vi "TW_Base64Conversion.vi"(9 "Base64 String in":string, 11 "String":string) -> (0 "error out":errorcluster, 1 "String out":string, 3 "Base64 String":string)   [LabVIEW 2019]
panel:
  in  "error in (no error)":errorcluster
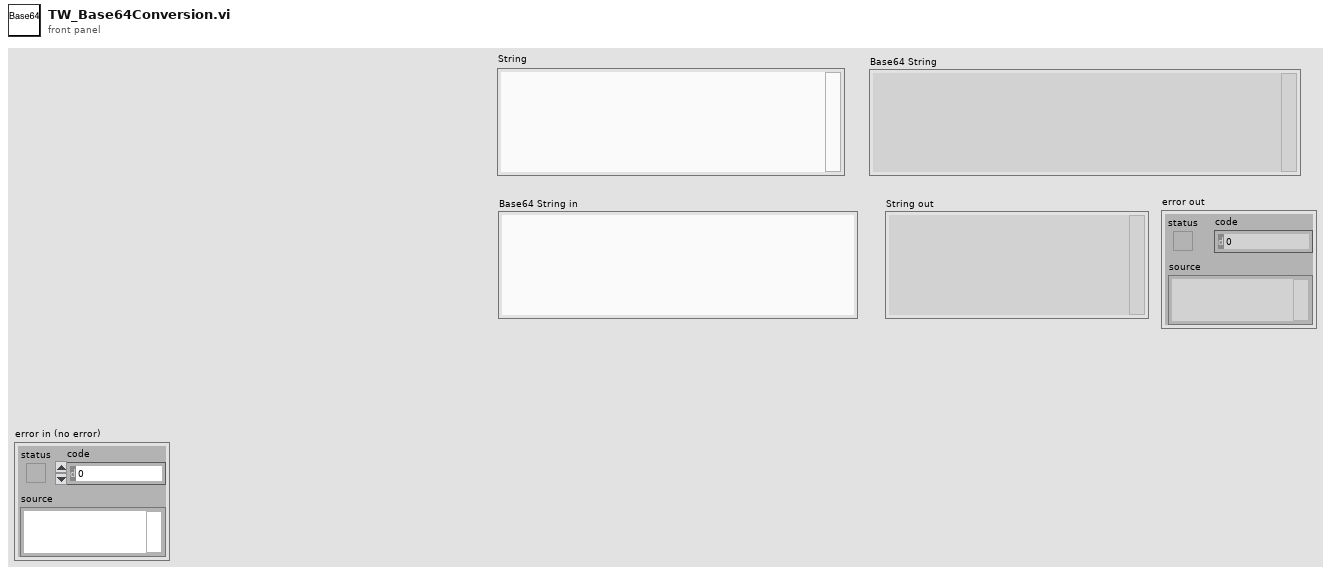
[diagram p1: front panel]
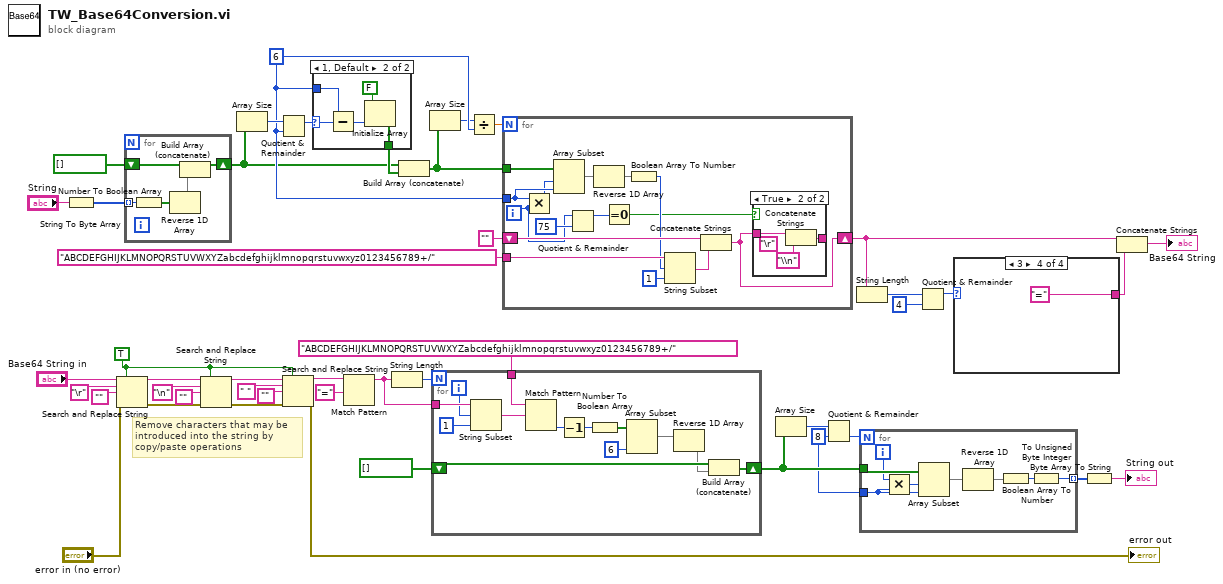
[diagram p0: block diagram]
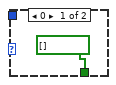
[diagram p2: hidden frame]
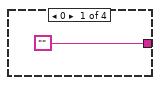
[diagram p3: hidden frame]
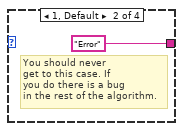
[diagram p4: hidden frame]
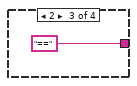
[diagram p5: hidden frame]
diagram:
  w1 = TRUE ("replace all? (F)")
  w18 = 8 ("y")
  w30 = 6 ("y")
  # "Remove characters that may be\nintroduced into the string by\ncopy/paste operations"
  n1 = String To Byte Array(string="String") -> (unsigned byte array=w44:u8[])
  n2 = Search and Replace String(replace all?=w1, input string="Base64 String in", search string="\r" ("replace string (\"\")"), replace string="", error in="error in (no error)") -> (result string=w11:string, error out=w9:errorcluster)  [unwired: 5 out]
  n3 = for {
    tunnel: w44 -> [w50] mode=indexing
    shift-right: [w47] -> w27
    shift-left: bool[] [] -> [w49]
    n4 = Number To Boolean Array(number=w50) -> (Boolean array=w48:bool[])
    n5 = Reverse 1D Array(array=w48) -> (reversed array=w46:bool[])
    n6 = Build Array (concatenate)(w49, w46) -> (w47:bool[])
  }
  n7 = Search and Replace String(replace all?=w1, input string=w11, search string="\n" ("replace string (\"\")"), replace string="", error in=w9) -> (result string=w5:string, error out=w4:errorcluster)  [unwired: 5 out]
  n8 = Array Size(array=w27) -> (size(s)=w33:i32)
  n9 = Quotient & Remainder(x=w33, y=w30) -> (x-y*floor(x/y)=w32:i32)  [unwired: 1 out]
  n10 = Search and Replace String(replace all?=w1, input string=w5, search string=" " ("replace string (\"\")"), replace string="", error in=w4) -> (result string=w2:string, error out=→"error out":errorcluster)  [unwired: 5 out]
  n11 = case shown="1, Default" w32 {
    selector: w32 -> [_ w55]
    tunnel: [bool[] [] w52] -> w31
    tunnel: w30 -> [_ w54]
    frame 0 {
    }
    frame 1, Default {
      n12 = Subtract(x=w54, y=w55) -> (x-y=w56:i32)
      n13 = Initialize Array(FALSE, w56) -> (w52:bool[])
    }
  }
  n14 = Match Pattern(string=w2, regular expression="=") -> (before substring=w23:string)  [unwired: 4 out]
  n15 = String Length(string=w23) -> (length=w26:i32)
  n16 = Build Array (concatenate)(w27, w31) -> (w29:bool[])
  n17 = Array Size(array=w29) -> (size(s)=w28:i32)
  n18 = for {
    N: w26 -> [_]
    tunnel: w23 -> [w69]
    tunnel: "ABCDEFGHIJKLMNOPQRSTUVWXYZabcdefghijklmnopqrstuvwxyz0123456789+/" -> [w66]
    shift-right: [w59] -> w19
    shift-left: bool[] [] -> [w58]
    i -> [w67]
    n19 = String Subset(string=w69, offset (0)=w67, length (rest)=1 ("length (rest)")) -> (substring=w65:string)
    n20 = Match Pattern(string=w66, regular expression=w65) -> (offset past match=w64:i32)  [unwired: 1 in, 3 out]
    n21 = Decrement(x=w64) -> (x-1=w63:i32)
    n22 = Number To Boolean Array(number=w63) -> (Boolean array=w62:bool[])
    n23 = Array Subset(array=w62, length=6) -> (w60:bool[])  [unwired: 1 in]
    n24 = Reverse 1D Array(array=w60) -> (reversed array=w57:bool[])
    n25 = Build Array (concatenate)(w58, w57) -> (w59:bool[])
  }
  n26 = Divide(x=w28, y=w30) -> (x/y=w34:dbl)
  n27 = for {
    N: w34 -> [_]
    tunnel: w29 -> [w84]
    tunnel: w30 -> [w83]
    tunnel: "ABCDEFGHIJKLMNOPQRSTUVWXYZabcdefghijklmnopqrstuvwxyz0123456789+/" -> [w82]
    shift-right: [w70] -> w36
    shift-left: "" -> [w80]
    i -> [w73]
    n28 = Multiply(x=w83, y=w73) -> (x*y=w74:i32)
    n29 = Array Subset(array=w84, index=w74, length=w83) -> (w76:bool[])
    n30 = Quotient & Remainder(x=w73, y=75) -> (x-y*floor(x/y)=w72:i32)  [unwired: 1 out]
    n31 = Reverse 1D Array(array=w76) -> (reversed array=w77:bool[])
    n32 = Equal To 0?(x=w72) -> (x = 0?=w71:bool)
    n33 = Boolean Array To Number(Boolean array=w77) -> (number=w78:u32)
    n34 = String Subset(string=w82, offset (0)=w78, length (rest)=1 ("length (rest)")) -> (substring=w79:string)
    n35 = Concatenate Strings(w80, w79) -> (w70:string)
    n36 = case shown="True" w71 {
      tunnel: w70 -> [w85 w87]
      tunnel: [w85 w88] -> _
      frame False {
      }
      frame True {
        (unwired) "\r"
        n37 = Concatenate Strings(w87, "\\n" ("string")) -> (w88:string)
      }
    }
  }
  n38 = Array Size(array=w19) -> (size(s)=w21:i32)
  n39 = Quotient & Remainder(x=w21, y=w18) -> (floor(x/y)=w20:i32)  [unwired: 1 out]
  n40 = String Length(string=w36) -> (length=w40:i32)
  n41 = for {
    N: w20 -> [_]
    tunnel: w19 -> [w96]
    tunnel: w18 -> [w95]
    tunnel: [w91] -> w17 mode=indexing
    i -> [w94]
    n42 = Multiply(x=w94, y=w95) -> (x*y=w89:i32)
    n43 = Array Subset(array=w96, index=w89, length=w95) -> (w93:bool[])
    n44 = Reverse 1D Array(array=w93) -> (reversed array=w90:bool[])
    n45 = Boolean Array To Number(Boolean array=w90) -> (number=w92:u32)
    n46 = To Unsigned Byte Integer(number=w92) -> (unsigned 8bit integer=w91:u8)
  }
  n47 = Quotient & Remainder(x=w40, y=4) -> (x-y*floor(x/y)=w38:i32)  [unwired: 1 out]
  n48 = case shown="3" w38 {
    tunnel: ["" "Error" "==" "="] -> w37
    frame 0 {
    }
    frame 1, Default {
      # "You should never\nget to this case. If\nyou do there is a bug\nin the rest of the algorithm."
    }
    frame 2 {
    }
    frame 3 {
    }
  }
  n49 = Byte Array To String(unsigned byte array=w17) -> (string=→"String out":string)
  n50 = Concatenate Strings(w36, w37) -> (→"Base64 String":string)
